vi "WriteDATAV2.vi"(8 "error in (no error)":errorcluster, 10 "Sample Name":string="TOKIN1", 11 "ChirpV2 in":refnum<class "ChirpV2.lvclass">) -> (0 "error out":errorcluster, 3 "ChirpV2 out":refnum<class "ChirpV2.lvclass">)   [LabVIEW 2014, in "ChirpV2.lvclass"]
uses:
  ChirpV2.lvclass
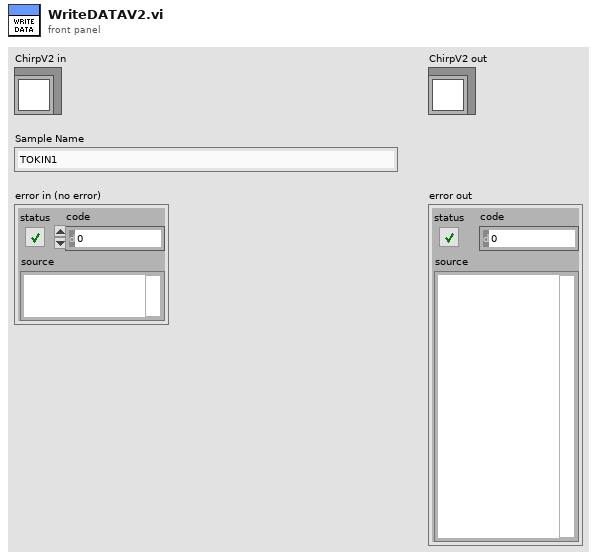
[diagram p1: front panel]
types:
  T1 = cluster{"exp_ID":i32, "Duration":dbl, "Rext":dbl, "Fstart":dbl, "Fend":dbl, "Fs":dbl, "Dc":dbl, "Window Ratio":dbl}
  T2 = cluster{"exp_ID":i32, "Time Stamp":timestamp, "sampleName":string}
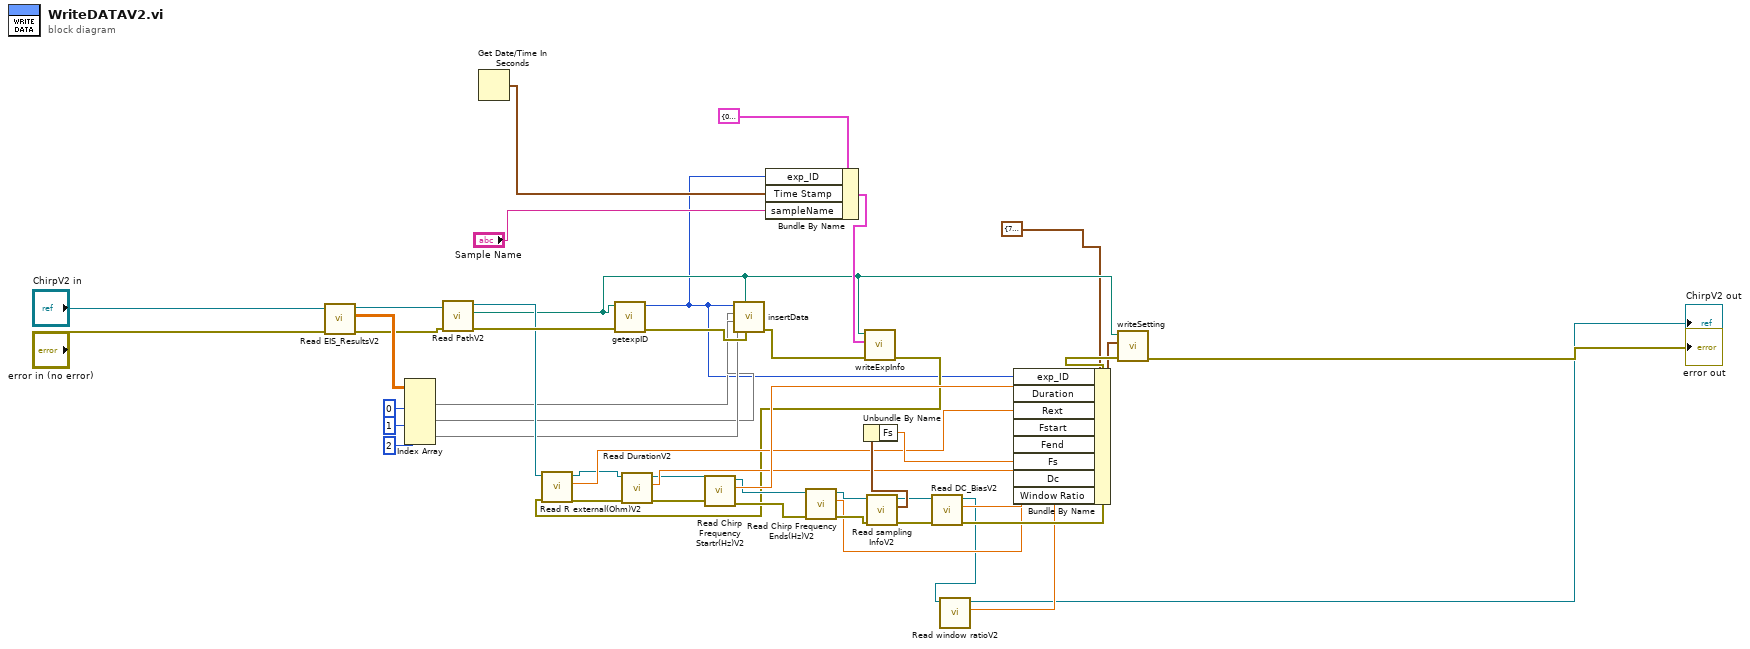
[diagram p0: block diagram]
diagram:
  n1 = call-dynamic "Read EIS_ResultsV2.vi"("error in (no error)"="error in (no error)", "ChirpV2 in"="ChirpV2 in") -> ("error out"=w9:errorcluster, "EIS_Results"=w13:dbl[][], "ChirpV2 out"=w8:refnum<class "ChirpV2.lvclass">)  [unwired: 7 in]
  n2 = Index Array(array=w13, index (col) #1=0 ("disabled index (col)"), index (col) #2=1 ("index (col)"), index (col) #3=2 ("index (col)")) -> (element #1=w14:dbl[], element #2=w15:dbl[], element #3=w16:dbl[])  [unwired: 3 in]
  n3 = call-dynamic "Read PathV2.vi"("error in (no error)"=w9, "ChirpV2 in"=w8) -> ("error out"=w44:errorcluster, "Path"=w18:path, "ChirpV2 out"=w43:refnum<class "ChirpV2.lvclass">)  [unwired: 7 in]
  n4 = Get Date/Time In Seconds() -> (seconds since 1Jan1904=w20:timestamp)
  n5 = call "getexpID.vi"("error in (no error)"=w44, "db_File"=w18) -> ("error out"=w17:errorcluster, "data"=w1:i32)  [unwired: 8 in]
  n6 = call "insertData.vi"("error in (no error)"=w17, "db_File"=w18, "P"=w16, "Z"=w15, "frequency"=w14, "exp_ID"=w1) -> ("error out"=w22:errorcluster)  [unwired: 5 in]
  n7 = Bundle By Name(cluster=T2 {"exp_ID"=0, "Time Stamp"=timestamp(0 s since 1904-01-01), "sampleName"=""} ("Exp_Info"), "exp_ID"=w1, "Time Stamp"=w20, "sampleName"="Sample Name") -> (w21:T2)
  n8 = call "writeExpInfo.vi"("error in (no error)"=w22, "Exp_Info"=w21, "db_File"=w18) -> ("error out"=w23:errorcluster)  [unwired: 8 in]
  n9 = call-dynamic "Read R external(Ohm)V2.vi"("error in (no error)"=w23, "ChirpV2 in"=w43) -> ("error out"=w25:errorcluster, "R external(Ohm)"=w26:dbl, "ChirpV2 out"=w24:refnum<class "ChirpV2.lvclass">)  [unwired: 7 in]
  n10 = call-dynamic "Read DurationV2.vi"("error in (no error)"=w25, "ChirpV2 in"=w24) -> ("error out"=w29:errorcluster, "Duration"=w28:dbl, "ChirpV2 out"=w27:refnum<class "ChirpV2.lvclass">)  [unwired: 7 in]
  n11 = call-dynamic "Read Chirp Frequency Startr(Hz)V2.vi"("error in (no error)"=w29, "ChirpV2 in"=w27) -> ("error out"=w32:errorcluster, "Chirp Frequency Startr(Hz)"=w31:dbl, "ChirpV2 out"=w30:refnum<class "ChirpV2.lvclass">)  [unwired: 7 in]
  n12 = call-dynamic "Read Chirp Frequency Ends(Hz)V2.vi"("error in (no error)"=w32, "ChirpV2 in"=w30) -> ("error out"=w35:errorcluster, "Chirp Frequency Ends(Hz)"=w34:dbl, "ChirpV2 out"=w33:refnum<class "ChirpV2.lvclass">)  [unwired: 7 in]
  n13 = call-dynamic "Read sampling InfoV2.vi"("error in (no error)"=w35, "ChirpV2 in"=w33) -> ("error out"=w39:errorcluster, "sampling Info"=w37:cluster{"Fs":dbl}, "ChirpV2 out"=w36:refnum<class "ChirpV2.lvclass">)  [unwired: 7 in]
  n14 = Unbundle By Name(w37) -> ("Fs"=w38:dbl)
  n15 = call-dynamic "Read DC_BiasV2.vi"("error in (no error)"=w39, "ChirpV2 in"=w36) -> ("error out"=w41:errorcluster, "DC_Bias"=w40:dbl, "ChirpV2 out"=w4:refnum<class "ChirpV2.lvclass">)  [unwired: 7 in]
  n16 = call-dynamic "Read window ratioV2.vi"("ChirpV2 in"=w4) -> ("window ratio"=w3:dbl, "ChirpV2 out"=→"ChirpV2 out":refnum<class "ChirpV2.lvclass">)  [unwired: 8 in, 1 out]
  n17 = Bundle By Name(cluster=T1 {"exp_ID"=72, "Duration"=50.0, "Rext"=33.0, "Fstart"=0.001, "Fend"=10.0, "Fs"=200.0, "Dc"=0.0, "Window Ratio"=0.0} ("eis_setting"), "exp_ID"=w1, "Duration"=w28, "Rext"=w26, "Fstart"=w31, "Fend"=w34, "Fs"=w38, "Dc"=w40, "Window Ratio"=w3) -> (w5:T1)
  n18 = call "writeSetting.vi"("error in (no error)"=w41, "eis_setting"=w5, "db_File"=w18) -> ("error out"=→"error out":errorcluster)  [unwired: 8 in]
